vi "AlazarSetTriggerDelay.vi"(3 "error in (no error)":errorcluster, 4 "Delay":u32, 5 "Handle":u64) -> (0 "error out":errorcluster, 1 "Return Code":u32, 2 "Handle":u64)   [LabVIEW 2018]
doc: "Set the time, in sample clocks, to wait after receiving a trigger event before capturing a record for the trigger."
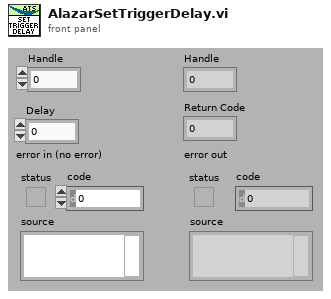
[diagram p1: front panel]
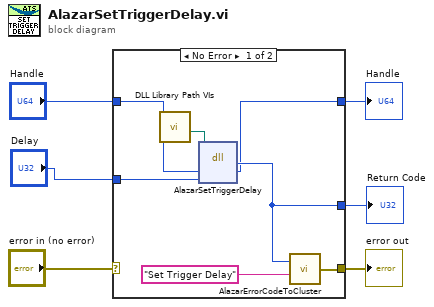
[diagram p0: block diagram]
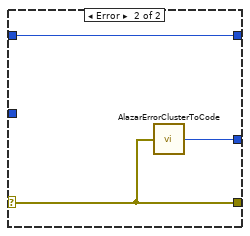
[diagram p2: hidden frame]
diagram:
  n1 = case shown="No Error" "error in (no error)" {
    selector: "error in (no error)" -> [_ w16]
    tunnel: [w10 w16] -> w5
    tunnel: [w12 w15] -> w4
    tunnel: "Handle" -> [w13 w14]
    tunnel: [w9 w14] -> w2
    tunnel: "Delay" -> [w8 _]
    frame No Error {
      n2 = call "DLL Library Path VIs.vi"() -> ("Alazar"=w7:path)  [unwired: 8 in, 3 out]
      n3 = dll-call lib="C:/Project/SerialSectOCT - FFT GPU/SerialSectOCT/Labview Software/DLL/ATSApi.dll" fn="AlazarSetTriggerDelay"(path in=w7, "handle"=w13, "value"=w8) -> ("return type"=w12:u32, "handle"=w9:u64)  [unwired: 3 in, 2 out]
      n4 = call "AlazarErrorCodeToCluster.vi"("Message"="Set Trigger Delay", "Error Code"=w12) -> ("error out"=w10:errorcluster)
    }
    frame Error {
      n5 = call "AlazarErrorClusterToCode.vi"("error in (no error)"=w16) -> ("Error Code"=w15:u32)
    }
  }
  "Handle" <- w2
  "error out" <- w5
  "Return Code" <- w4
